vi "display_environ (SubVI).vi"(11 "environ cluster":cluster{dbl[], dbl[]}) -> (0 "P_pirani":dbl, 1 "P_cc":dbl, 2 "T_opt_table":dbl, 3 "T_elec_rack":dbl, 4 "P_baratron":dbl)   [LabVIEW 2018]
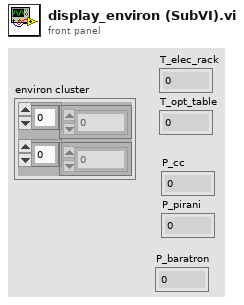
[diagram p1: front panel]
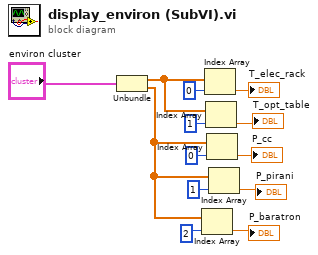
[diagram p0: block diagram]
diagram:
  n1 = Unbundle("environ cluster") -> (w9:dbl[], w1:dbl[])
  n2 = Index Array(array=w1, index=2) -> (element=→"P_baratron":dbl)
  n3 = Index Array(array=w9, index=0) -> (element=→"T_elec_rack":dbl)
  n4 = Index Array(array=w9, index=1) -> (element=→"T_opt_table":dbl)
  n5 = Index Array(array=w1, index=0) -> (element=→"P_cc":dbl)
  n6 = Index Array(array=w1, index=1) -> (element=→"P_pirani":dbl)
